vi "BRig_RT__Case_Exp__storeData__endExp__v5__p2.vi"(0 "input_dataCurrent":u16[](array[numeric]), 1 "input_dataLick":u16[][](array[numeric]), 7 "input_True":bool=TRUE, 11 "input_dataMTrig":u16[](array[numeric])) -> (8 "output_True":bool)   [LabVIEW 2014]
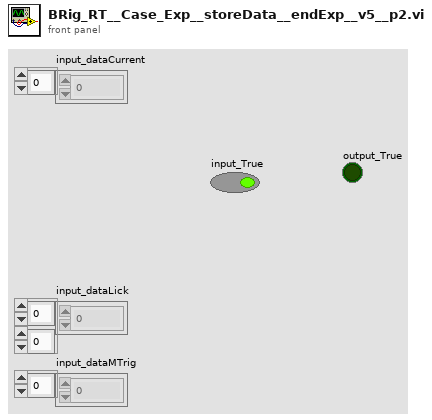
[diagram p1: front panel]
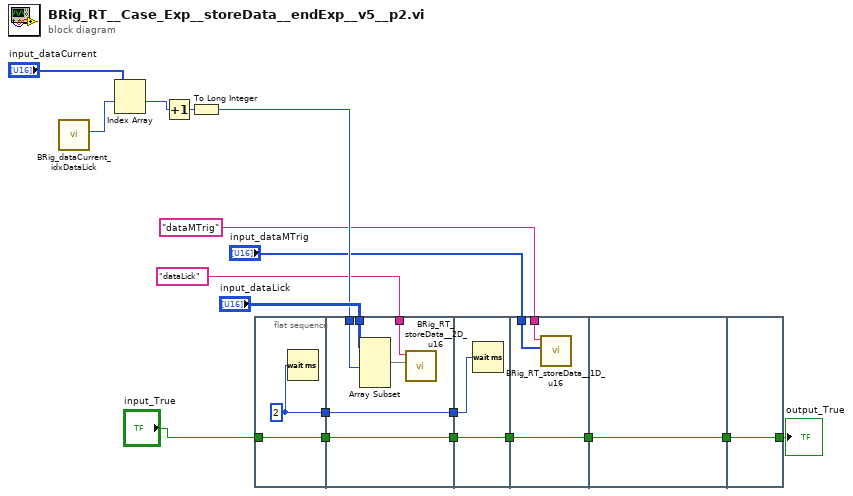
[diagram p0: block diagram]
diagram:
  n1 = call "BRig_dataCurrent_idxDataLick.vi"() -> ("output_idxDataLick"=w12:i32)  [unwired: 11 in]
  n2 = Index Array(array="input_dataCurrent", index #1=w12) -> (element #1=w11:u16)  [unwired: 1 in, 1 out]
  n3 = Increment(x=w11) -> (x+1=w10:u16)
  n4 = To Long Integer(number=w10) -> (32bit integer=w16:i32)
  n5 = flat-sequence {
    tunnel: [w20] -> w6
    tunnel: "input_True" -> [w20]
    tunnel: [w19] -> w2
    tunnel: "input_dataLick" -> [w26]
    tunnel: w16 -> [w25]
    tunnel: "dataLick" ("input_filename") -> [w23]
    tunnel: [w22] -> w4
    tunnel: w6 -> [w22]
    tunnel: w2 -> [w21]
    tunnel: [w21] -> w1
    tunnel: w4 -> [w28]
    tunnel: [w28] -> w3
    tunnel: w1 -> [w27]
    tunnel: "input_dataMTrig" -> [w31]
    tunnel: "dataMTrig" ("input_filename") -> [w30]
    tunnel: [w29] -> w8
    tunnel: w3 -> [w29]
    tunnel: [w32] -> w9
    tunnel: w8 -> [w32]
    tunnel: [w33] -> w7
    tunnel: w9 -> [w33]
    frame #0 {
      w19 = u32 2 ("milliseconds to wait")
      n6 = Wait (ms)(milliseconds to wait=w19) -> ()  [unwired: 1 out]
    }
    frame #1 {
      n7 = Array Subset(array=w26, length (row)=w25) -> (w24:u16[][])  [unwired: 3 in]
      n8 = call "BRig_RT_storeData__2D_u16.vi"("Array"=w24, "input_filename"=w23) -> ()  [unwired: 10 in]
    }
    frame #2 {
      n9 = Wait (ms)(milliseconds to wait=w27) -> ()  [unwired: 1 out]
    }
    frame #3 {
      n10 = call "BRig_RT_storeData__1D_u16.vi"("Array"=w31, "input_filename"=w30) -> ()  [unwired: 10 in]
    }
    frame #4 {
    }
    frame #5 {
    }
  }
  "output_True" <- w7
